vi "Find Largest Image.vi"(10 "Images":refnum<class "SVGImage.lvclass">[](array[class])) -> (2 "Largest Image":refnum<class "SVGImage.lvclass">)   [LabVIEW 2019, in "SVGImage.lvclass"]
uses:
  SVGImage.lvclass
  SVGImage.lvclass/SVGImage.ctl
  Read Height.vi
  Read Width.vi
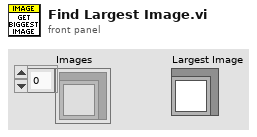
[diagram p1: front panel]
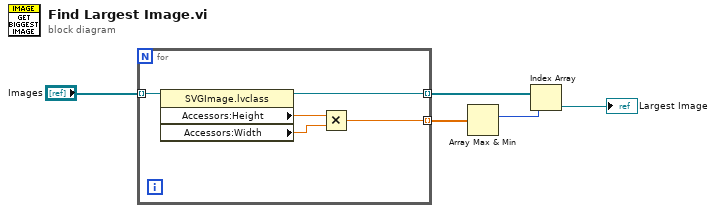
[diagram p0: block diagram]
diagram:
  n1 = for {
    tunnel: "Images" -> [w10] mode=indexing
    tunnel: [w6] -> w4 mode=indexing
    tunnel: [w9] -> w5 mode=indexing
    n2 = property class="SVGImage.lvclass"(reference=w10) -> (reference out=w9:refnum<class "SVGImage.lvclass">, "Accessors:Height"=w8:dbl, "Accessors:Width"=w7:dbl)  [unwired: 1 in, 1 out]
    n3 = Multiply(x=w8, y=w7) -> (x*y=w6:dbl)
  }
  n4 = Array Max & Min(array=w4) -> (max index (indices)=w3:i32)  [unwired: 3 out]
  n5 = Index Array(array=w5, index=w3) -> (element=→"Largest Image":refnum<class "SVGImage.lvclass">)
